vi "Init Core.vi"(8 "error in (no error)":errorcluster, 11 "Module in":refnum<class "Module.lvclass">) -> (0 "error out":errorcluster, 3 "Module out":refnum<class "Module.lvclass">)   [LabVIEW 2020, in "Volatus.lvlib" / "Module.lvclass"]
uses:
  Module.lvclass
  State.ctl
  Module.lvclass/Module.ctl
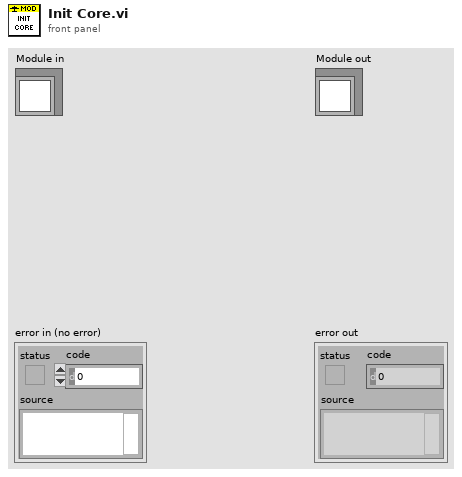
[diagram p1: front panel]
types:
  T1 = typedef "Volatus.lvlib/Module.lvclass/State.ctl" = enum16{"Unknown", "Launched", "Starting", "Running", "Stopping", "Stopped", "Error - Starting", "Error - Run", "Error - Stopping"}
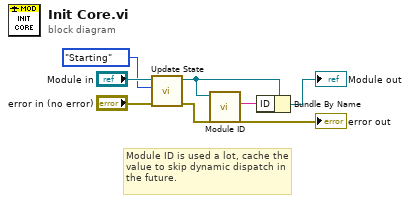
[diagram p0: block diagram]
diagram:
  # "Module ID is used a lot, cache the value to skip dynamic dispatch in the future."
  n1 = call "Update State.vi"("error in (no error)"="error in (no error)", "State"=State."Starting", "Module in"="Module in") -> ("error out"=→"error out":errorcluster, "Module out"=w4:refnum<class "Module.lvclass">)  [unwired: 7 in]
  n2 = call-dynamic "Module ID.vi"("Module in"=w4) -> ("Module ID"=w3:string)  [unwired: 10 in]
  n3 = Bundle By Name(cluster=w4, "ID"=w3) -> (→"Module out":refnum<class "Module.lvclass">)
